vi "Ex1_BooleanCaseStructure.vi"() -> ()   [LabVIEW 2024]
panel:
  in  "OK Button":bool
  in  "OK Button 2":bool
  out "Numeric 3":dbl
  in  "Numeric 2":dbl
  in  "Numeric":dbl
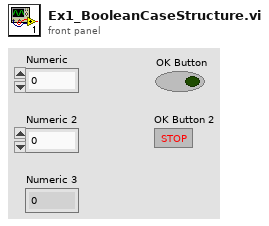
[diagram p1: front panel]
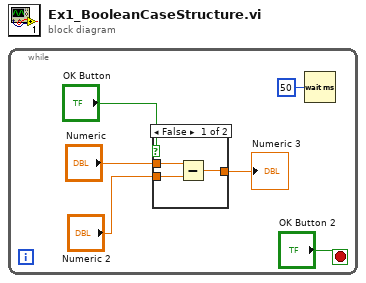
[diagram p0: block diagram]
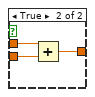
[diagram p2: hidden frame]
diagram:
  n1 = while {
    stop <- "OK Button 2" stop-if-true
    n2 = case shown="False" "OK Button" {
      tunnel: "Numeric 2" -> [w7 w12]
      tunnel: "Numeric" -> [w8 w11]
      tunnel: [w9 w10] -> w4
      frame False {
        n3 = Subtract(x=w8, y=w7) -> (x-y=w9:dbl)
      }
      frame True {
        n4 = Add(x=w11, y=w12) -> (x+y=w10:dbl)
      }
    }
    "Numeric 3" <- w4
    n5 = Wait (ms)(milliseconds to wait=u32 50) -> ()  [unwired: 1 out]
  }
